vi "Sensor Bits To String.vi"(8 "error in (no error)":errorcluster caption="错误输入（无错误）", 9 "BitBufferSize":i32, 10 "pszSourceBuffer":string, 11 "sensorHandle":i32) -> (0 "error out":errorcluster caption="错误输出", 2 "pszSourceBuffer out":string, 3 "function return":i32)   [LabVIEW 2020]
doc: "extern int __stdcall APSxSensorBitsToString (int sensorHandle, OUT char pszSourceBuffer[], IN int BitBufferSize);"
uses:
  APSx.dll/APSx.dll
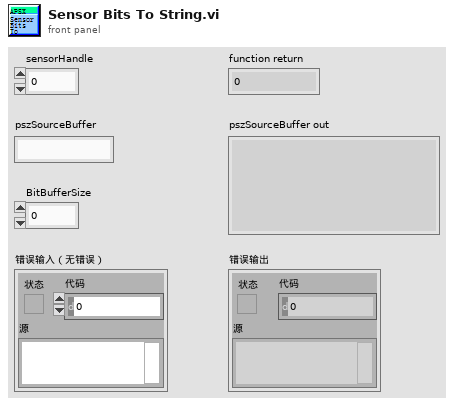
[diagram p1: front panel]
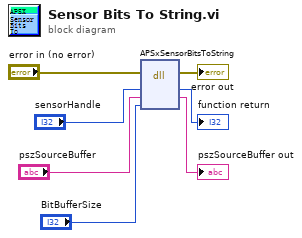
[diagram p0: block diagram]
diagram:
  n1 = dll-call lib="PTH2gabs CUsersFengDesktop传感器对中台传感器对中台labviewSourcesAPSx.dllAPSx.*" fn="APSxSensorBitsToString"(error in="error in (no error)", "sensorHandle"="sensorHandle", "pszSourceBuffer"="pszSourceBuffer", "BitBufferSize"="BitBufferSize") -> (error out=→"error out":errorcluster, "sensorHandle"=→"function return":i32, "pszSourceBuffer"=→"pszSourceBuffer out":string)  [unwired: 4 in, 1 out]
